vi "2016-120_Initialize PS.vi"(6 "Current Limit (0)":dbl=3.0 min=0.0 max=6.0 format="%#.2g", 8 "error in":errorcluster, 9 "Output Voltage (0)":dbl min=0.0 max=18.0 format="%#.2f", 10 "Maximum Output Voltage (18)":dbl=32.0 min=0.0 max=72.0 format="%#.2f", 11 "Port":i32) -> (0 "error out":errorcluster, 3 "VISA resource name out":refnum<visa-resource-name>="COM7")   [LabVIEW 2015]
uses:
  <instrlib>/BK Precision 178XB Series/BK Precision 178XB Series.lvlib
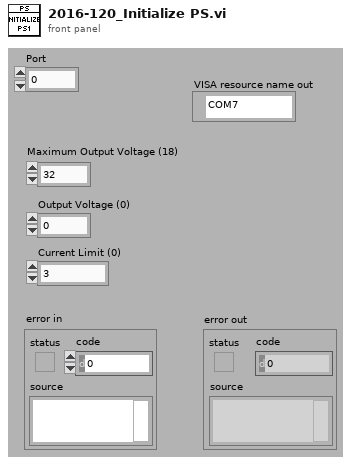
[diagram p1: front panel]
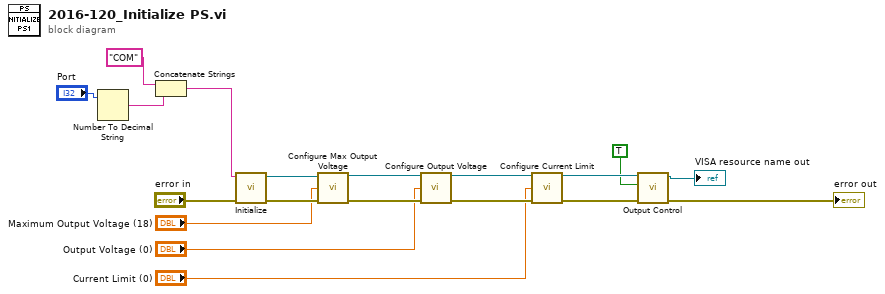
[diagram p0: block diagram]
diagram:
  n1 = Number To Decimal String(number="Port") -> (decimal integer string=w2:string)  [unwired: 1 in]
  n2 = Concatenate Strings("COM" ("string"), w2) -> (w3:string)
  n3 = call "Initialize.vi"("error in (no error)"="error in", "VISA resource name"=w3) -> ("error out"=w17:errorcluster, "VISA resource name out"=w18:refnum<visa-resource-name>)  [unwired: 8 in]
  n4 = call "Configure Max Output Voltage.vi"("VISA resource name"=w18, "Maximum Output Voltage (18)"="Maximum Output Voltage (18)", "error in (no error)"=w17) -> ("VISA resource name out"=w16:refnum<visa-resource-name>, "error out"=w13:errorcluster)  [unwired: 11 in]
  n5 = call "Configure Output Voltage.vi"("VISA resource name"=w16, "Output Voltage (0)"="Output Voltage (0)", "error in (no error)"=w13) -> ("VISA resource name out"=w15:refnum<visa-resource-name>, "error out"=w14:errorcluster)  [unwired: 11 in]
  n6 = call <instrlib>:"Configure Current Limit.vi"("VISA resource name"=w15, "Current Limit (0)"="Current Limit (0)", "error in (no error)"=w14) -> ("VISA resource name out"=w12:refnum<visa-resource-name>, "error out"=w11:errorcluster)  [unwired: 11 in]
  n7 = call <instrlib>:"Output Control.vi"("error in (no error)"=w11, "Enable Output Terminals (F: Off)"=TRUE, "VISA resource name"=w12) -> ("error out"=→"error out":errorcluster, "VISA resource name out"=→"VISA resource name out":refnum<visa-resource-name>)  [unwired: 7 in]
